vi "RT_NetStreams.vi"() -> ()   [LabVIEW 2019]
panel:
  out "Sine1":dbl[](graph)
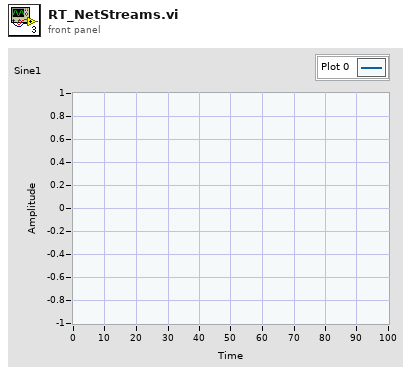
[diagram p1: front panel]
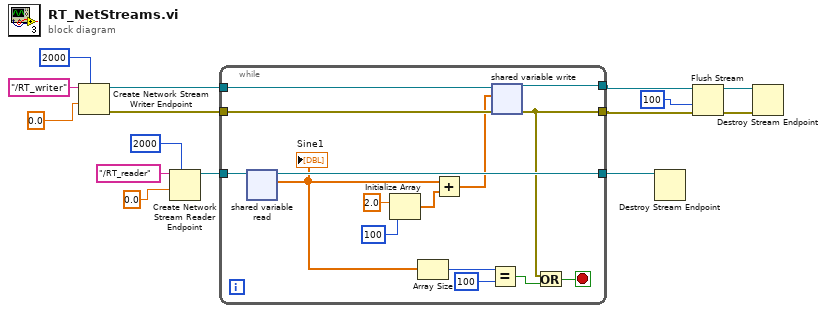
[diagram p0: block diagram]
diagram:
  n1 = Create Network Stream Writer Endpoint(7:2000 ("writer buffer size"), 9:0.0, 11:"/RT_writer" ("writer name")) -> (0:w7:errorcluster, 3:w8:refnum<k21>)  [unwired: 4 in]
  n2 = Create Network Stream Reader Endpoint(7:2000 ("reader buffer size"), 9:0.0, 11:"/RT_reader" ("reader name")) -> (3:w9:refnum<k21>)  [unwired: 4 in, 1 out]
  n3 = while {
    tunnel: [w30] -> w4
    tunnel: w8 -> [w24]
    tunnel: [w25] -> w2
    tunnel: w7 -> [w26]
    tunnel: [w21] -> w3
    tunnel: w9 -> [w29]
    stop <- w23 stop-if-true
    n4 = shared-variable-read(w29) -> (w30:refnum<k21>, w16:dbl[])  [unwired: 3 in, 2 out]
    "Sine1" <- w16
    n5 = Initialize Array(2.0 ("element"), 100 ("dimension size")) -> (w18:dbl[])
    n6 = Array Size(array=w16) -> (size(s)=w28:i32)
    n7 = Add(x=w16, y=w18) -> (x+y=w17:dbl[])
    n8 = Equal?(x=w28, y=100) -> (x = y?=w22:bool)
    n9 = shared-variable-write(w24, w26, w17) -> (w25:refnum<k21>, w21:errorcluster)  [unwired: 1 in, 1 out]
    n10 = Or(x=w21, y=w22) -> (x .or. y?=w23:bool)
  }
  n11 = Destroy Stream Endpoint(11:w4) -> ()  [unwired: 1 in, 1 out]
  n12 = Flush Stream(8:w3, 9:100 ("timeout in ms (-1)"), 11:w2) -> (0:w6:errorcluster, 3:w5:refnum<k21>)  [unwired: 1 in, 1 out]
  n13 = Destroy Stream Endpoint(8:w6, 11:w5) -> ()  [unwired: 1 out]
